vi "Queue FGV.vi"(7 "States":T1, 8 "error in (no error)":errorcluster, 11 "Message Q In":refnum<queue>) -> (0 "error out":errorcluster, 3 "Message Q Out":refnum<queue>)   [LabVIEW 2017, in "Messaging Library.lvlib"]
uses:
  Messaging Library.lvlib
  Controls/Q FGV States.ctl
  Controls/Msg TypeDef.ctl
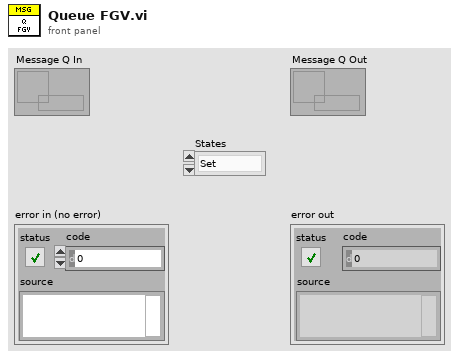
[diagram p1: front panel]
types:
  T1 = typedef "Messaging Library.lvlib/Q FGV States.ctl" = enum16{"Set", "Get"}
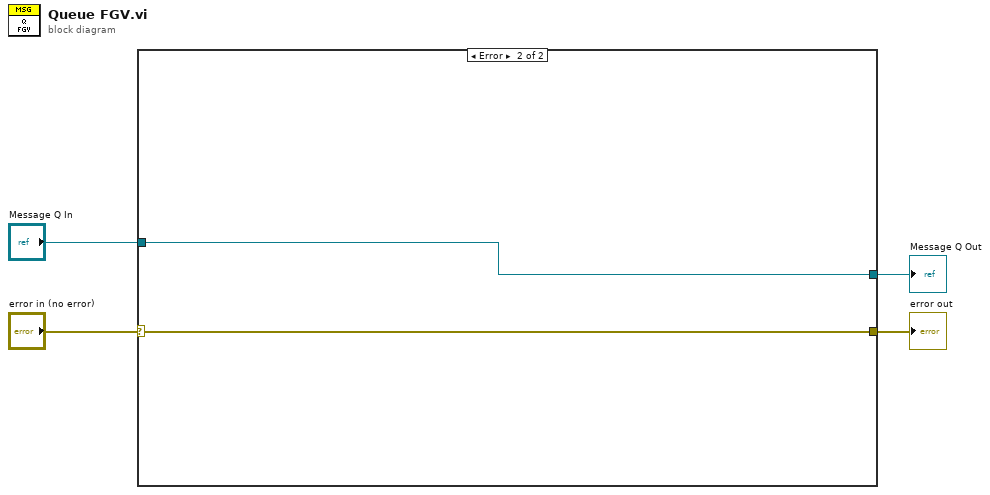
[diagram p0: block diagram]
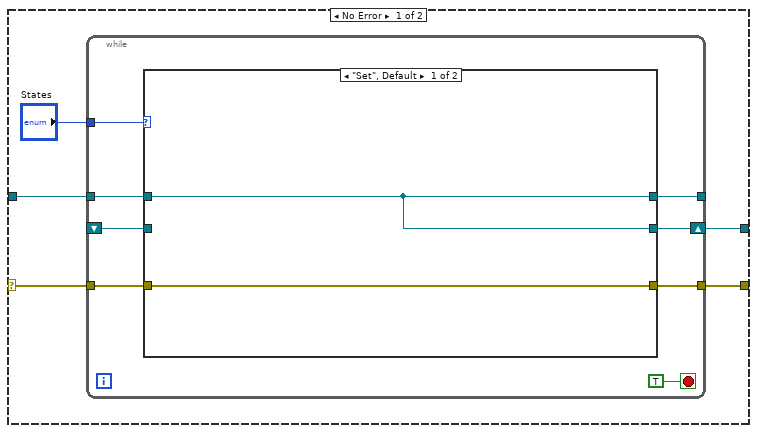
[diagram p2: hidden frame]
diagram:
  n1 = case shown="Error" "error in (no error)" {
    selector: "error in (no error)" -> [w9 w24]
    tunnel: [w5 w24] -> w3
    tunnel: "Message Q In" -> [w7 w23]
    tunnel: [w6 w23] -> w1
    frame No Error {
      n2 = while {
        tunnel: w9 -> [w16]
        tunnel: "States" -> [w15]
        tunnel: w7 -> [w14]
        tunnel: [w13] -> _
        shift-right: [w12] -> w6
        shift-left: _ -> [w11]
        tunnel: [w10] -> w5
        stop <- TRUE stop-if-true
        n3 = case shown="\"Set\", Default" w15 {
          tunnel: w16 -> [w18 w20]
          tunnel: w14 -> [w19 w22]
          tunnel: [w19 w22] -> w13
          tunnel: [w19 w21] -> w12
          tunnel: w11 -> [_ w21]
          tunnel: [w18 w20] -> w10
          frame "Set", Default {
          }
          frame "Get" {
          }
        }
      }
    }
    frame Error {
    }
  }
  "error out" <- w3
  "Message Q Out" <- w1
